vi "Write Value.vi"(7 "GPIO":refnum<class "GPIO.lvclass">, 8 "error in (no error)":errorcluster, 10 "Value":bool, 11 "Session In":refnum<class "Session.lvclass">) -> (0 "error out":errorcluster, 3 "Session Out":refnum<class "Session.lvclass">)   [LabVIEW 2020, in "CTI.lvlib" / "GPIO.lvclass"]
uses:
  GPIO.lvclass
  GPIO.lvclass/GPIO.ctl
  Session/Session.lvclass
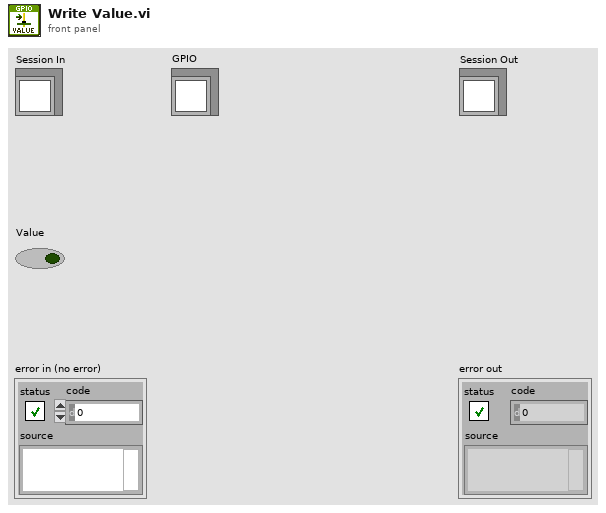
[diagram p1: front panel]
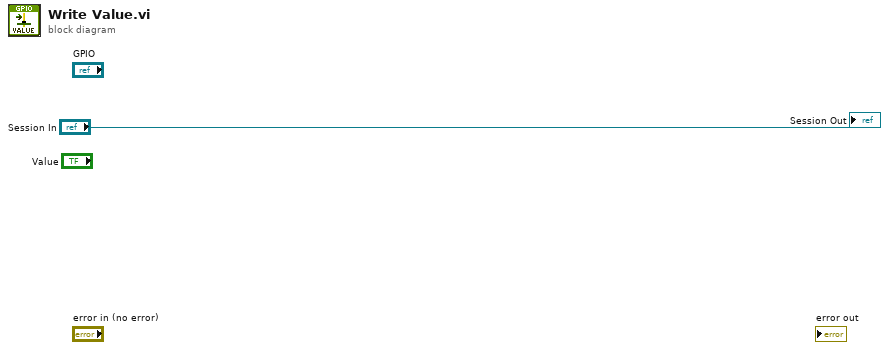
[diagram p0: block diagram]
diagram:
  "Session Out" <- "Session In"
